vi "Day 5 Mini UI and Type Calibration.vi"() -> ()   [LabVIEW 2026]
panel:
  out "OUTPUT -  FLOAT 3":dbl
  in  "INPUT - FLOAT 3":dbl
  out "OUTPUT - INT 2":i32
  in  "INPUT - INT 1":i32
  out "OUTPUT - INT":i32
  in  "INPUT - FLOAT":dbl
  # "Representing a Coertion Dot"
  # "Fixing a Coertion Dot by using representations\n to convert them to their matching Numeric type"
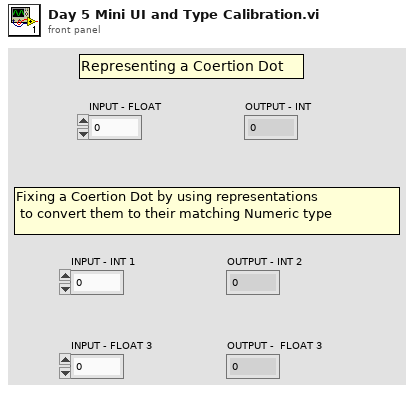
[diagram p1: front panel]
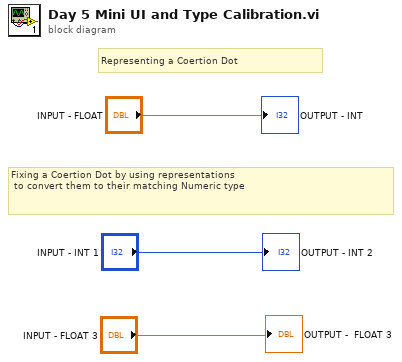
[diagram p0: block diagram]
diagram:
  # "Fixing a Coertion Dot by using representations\n to convert them to their matching Numeric type"
  # "Representing a Coertion Dot"
  "OUTPUT - INT" <- "INPUT - FLOAT"
  "OUTPUT - INT 2" <- "INPUT - INT 1"
  "OUTPUT -  FLOAT 3" <- "INPUT - FLOAT 3"
